vi "Register Verbose Explanation.vi"(7 "Unique Test ID":string, 8 "error in (no error)":errorcluster, 9 "Explanation":string, 10 "Unique Assert ID":string, 11 "Basic Test Manager in":refnum<class "Basic Test Manager.lvclass">) -> (0 "error out":errorcluster, 3 "Basic Test Manager out":refnum<class "Basic Test Manager.lvclass">)   [LabVIEW 2013, in "Caraya.lvlib" / "Basic Test Manager.lvclass"]
uses:
  Basic Test Manager.lvclass
  Test Result/Test Event Data.ctl
  Test Result/Test Verbose Explanation.ctl
  Basic Test Manager.lvclass/Basic Test Manager.ctl
  Test Result/Test Result.lvclass
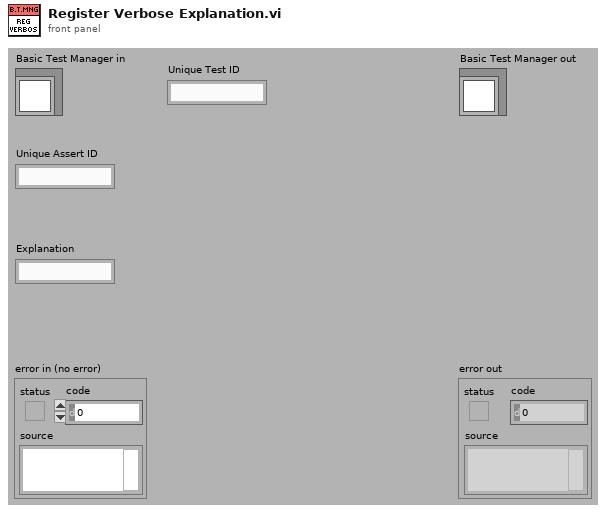
[diagram p1: front panel]
types:
  T1 = typedef "Caraya.lvlib/Test Result.lvclass/Test Verbose Explanation.ctl" = cluster{"Unique Test ID":string, "Unique Assert ID":string, "Explanation":string}
  T2 = typedef "Caraya.lvlib/Test Result.lvclass/Test Event Data.ctl" = cluster{"Label":string, "Argument":variant}
  T3 = typedef "Caraya.lvlib/Test Result.lvclass/Test Event.ctl" = refnum<user-event>
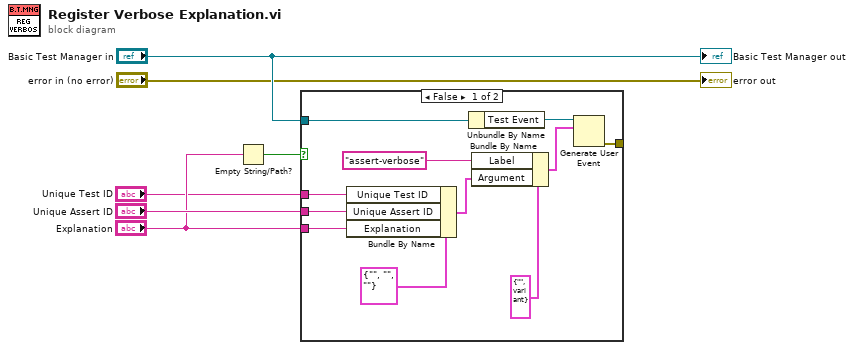
[diagram p0: block diagram]
diagram:
  n1 = Empty String/Path?(string/path="Explanation") -> (empty?=w4:bool)
  n2 = case shown="False" w4 {
    tunnel: "Basic Test Manager in" -> [w13 _]
    tunnel: "Unique Assert ID" -> [w10 _]
    tunnel: "Explanation" -> [w9 _]
    tunnel: [w8 _] -> _
    tunnel: "Unique Test ID" -> [w7 _]
    frame False {
      n3 = Bundle By Name(cluster=T1 {"Unique Test ID"="", "Unique Assert ID"="", "Explanation"=""} ("Verbose"), "Unique Test ID"=w7, "Unique Assert ID"=w10, "Explanation"=w9) -> (w11:T1)
      n4 = Unbundle By Name(w13) -> ("Test Event"=w17:T3)
      n5 = Bundle By Name(cluster=T2 {"Label"="", "Argument"=variant} ("Test Event"), "Label"="assert-verbose" ("Message"), "Argument"=w11) -> (w16:T2)
      n6 = Generate User Event(user event=w17, event data cluster=w16) -> (error out=w8:errorcluster)  [unwired: 2 in, 1 out]
    }
    frame True {
    }
  }
  "error out" <- "error in (no error)"
  "Basic Test Manager out" <- "Basic Test Manager in"
